vi "is_createdFromFactory.vi"(0 "HGF_Factory":refnum<class "HGF_Factory.lvclass">, 5 "error in (no error)":errorcluster) -> (14 "dup HGF_Factory":refnum<class "HGF_Factory.lvclass">, 16 "createdFromFactory?":bool, 19 "error out":errorcluster)   [LabVIEW 2014, in "HGF_BaseClasses.lvlib" / "HGF_Factory.lvclass"]
doc: "This VI returns a flag that indicates whether the object was created from a HGF_Factory or not."
uses:
  HGF_Factory.lvclass
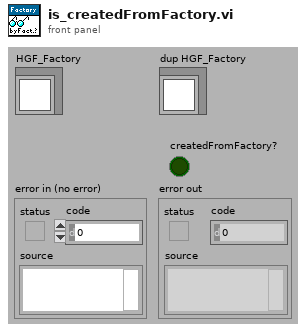
[diagram p1: front panel]
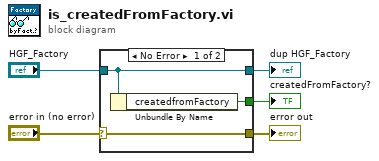
[diagram p0: block diagram]
diagram:
  n1 = case shown="No Error" "error in (no error)" {
    selector: "error in (no error)" -> [w8 w9]
    tunnel: [w8 w9] -> w4
    tunnel: [w7 w10] -> w2
    tunnel: "HGF_Factory" -> [w7 w10]
    tunnel: [w6 _] -> w1
    frame No Error {
      n2 = Unbundle By Name(w7) -> ("createdfromFactory"=w6:bool)
    }
    frame Error {
    }
  }
  "error out" <- w4
  "dup HGF_Factory" <- w2
  "createdFromFactory?" <- w1
